vi "采集正在进行.vi"() -> ()   [LabVIEW 2013]
panel:
  in  "采集正在进行":bool
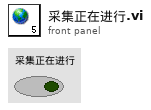
[diagram p1: front panel]
diagram:
